vi "Debug Global.vi"() -> ()   [LabVIEW 2017, in "FPGA-SRL.lvlib"]
uses:
  FPGA-SRL.lvlib
panel:
  out "Sim Write Memory":u16[](array[numeric]) format="%08x"
  in  "CH (1-24)":i32
  in  "DIN":bool
  in  "SYNC":bool
  in  "SCLK":bool
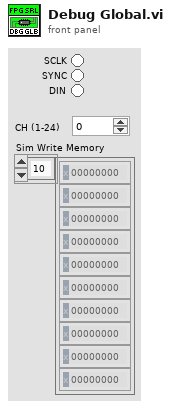
[diagram p1: front panel]
diagram:
